vi "Field_Calc_Ball_Pixel_Location.vi"(4 "Y Conv":dbl, 6 "X Conv":dbl, 9 "Y  INCHES - BALL":dbl, 11 "X INCHES - BALL":dbl) -> (1 "Top Pixel":dbl, 3 "Left Pixel":dbl)   [LabVIEW 2019]
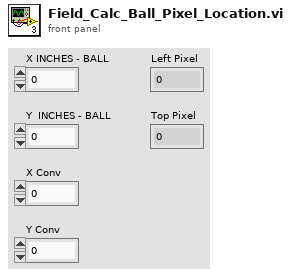
[diagram p1: front panel]
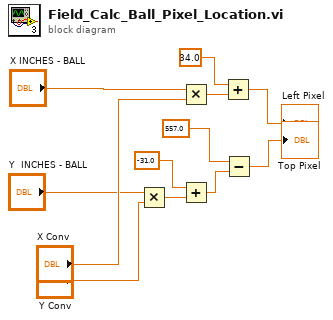
[diagram p0: block diagram]
diagram:
  n1 = Multiply(x="Y  INCHES - BALL", y="Y Conv") -> (x*y=w4:dbl)
  n2 = Multiply(x="X INCHES - BALL", y="X Conv") -> (x*y=w1:dbl)
  n3 = Add(x=-31.0, y=w4) -> (x+y=w7:dbl)
  n4 = Add(x=34.0, y=w1) -> (x+y=→"Left Pixel":dbl)
  n5 = Subtract(x=557.0, y=w7) -> (x-y=→"Top Pixel":dbl)
